vi "sub build b data.vi"(8 "error in":errorcluster, 11 "<b> data":T1) -> (0 "error out":errorcluster, 3 "<b> string":string)   [LabVIEW 2018, in "Data Parser.lvclass"]
uses:
  Data Parser.lvclass
  frame b data.ctl
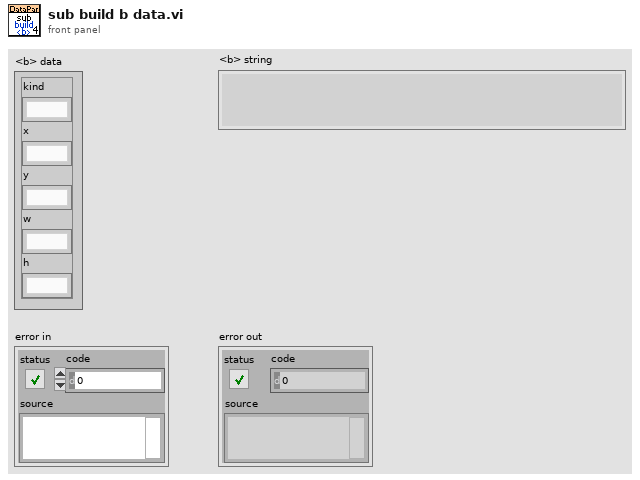
[diagram p1: front panel]
types:
  T1 = typedef "Data Parser.lvclass/frame b data.ctl" = cluster{"kind":string, "x":string, "y":string, "w":string, "h":string}
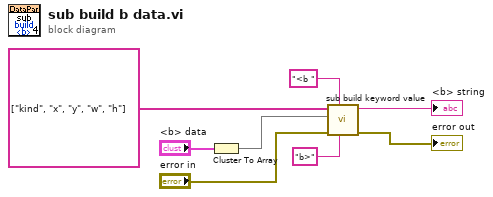
[diagram p0: block diagram]
diagram:
  n1 = Cluster To Array(cluster="<b> data") -> (array=w7:string[])
  n2 = call "sub build keyword value.vi"("EOF"="b>" ("SOF"), "SOF"="<b ", "error in"="error in", "value"=w7, "keyword"=string[] ["kind", "x", "y", "w", "h"]) -> ("error out"=→"error out":errorcluster, "keyword value string"=→"<b> string":string)  [unwired: 5 in]
